vi "Open Receiver UDP Connection.vi"(4 "Multicast Address":string="234.5.6.7", 5 "Port":i32=3456) -> (0 "error out":errorcluster, 2 "UDP Network Connection Refnum":refnum<k16>)   [LabVIEW 2013]
uses:
  subVIs.llb/UDP Multicast Open.vi
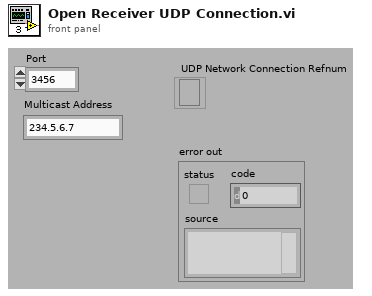
[diagram p1: front panel]
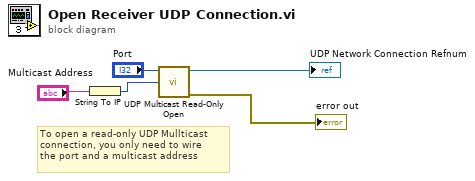
[diagram p0: block diagram]
diagram:
  # "To open a read-only UDP Mullticast\nconnection, you only need to wire\nthe port and a multicast address"
  n1 = String To IP(1:"Multicast Address") -> (0:w5:u32)
  n2 = call-poly "UDP Multicast Read-Only Open.vi"("multicast addr"=w5, "port"="Port") -> ("error out"=→"error out":errorcluster, "connection ID"=→"UDP Network Connection Refnum":refnum<k16>)  [unwired: 1 in, 7 out]
